vi "PicoScope3000aGetStreamingValues.vi"(9 "deviceIndex":u16, 11 "error in":errorcluster) -> (0 "Start Index":u32, 1 "Trigger":cluster{bool, "triggeredAt (Total samples)":u32}, 3 "error out":errorcluster, 4 "Number of Samples":i32, 5 "ready":i16, 6 "Auto Stopped":bool)   [LabVIEW 2010]
doc: "This VI is used in streaming mode to get the latest values from the driver. It should be called in a loop after the oscilloscope has been set up using PicoScope3000aSettings.vi and streaming has been started by calling PicoScope3000aStartStreaming.vi. The VI outputs the number of samples available and the start index of these samples in the array output by PicoScope3000aStartStreaming.vi."
uses:
  ps3000aWrap.dll
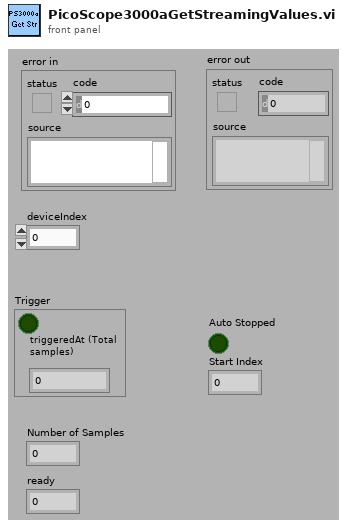
[diagram p1: front panel]
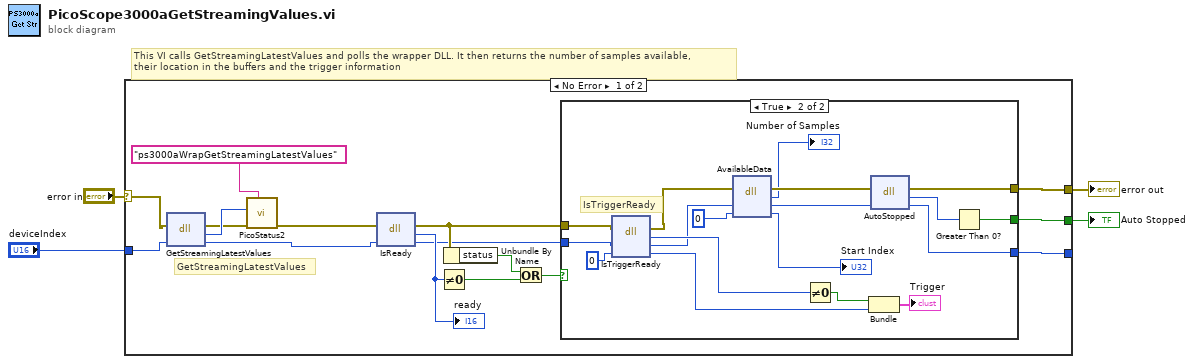
[diagram p0: block diagram]
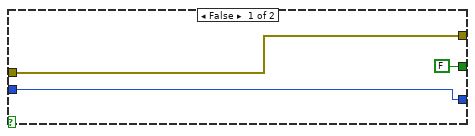
[diagram p2: hidden frame]
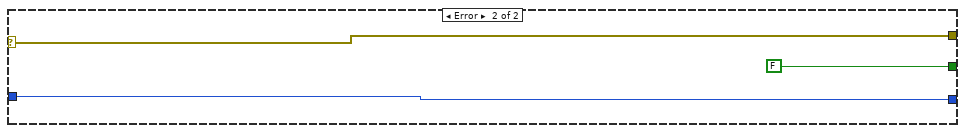
[diagram p3: hidden frame]
diagram:
  # "This VI calls GetStreamingLatestValues and polls the wrapper DLL. It then returns the number of samples available, \ntheir location in the buffers and the trigger information"
  n1 = case shown="No Error" "error in" {
    selector: "error in" -> [w14 w44]
    tunnel: [w20 w44] -> w3
    tunnel: [w19 w42] -> _
    tunnel: [w18 FALSE] -> w2
    tunnel: "deviceIndex" -> [w9 w42]
    frame No Error {
      # "GetStreamingLatestValues"
      n2 = dll-call lib="ps3000aWrap.dll" fn="GetStreamingLatestValues" ("PS5000.dll:_ps5000SetDataBuffer@16")(error in=w14, "deviceIndex"=w9) -> (error out=w7:errorcluster, "PICO_STATUS"=w8:u32, "deviceIndex"=w13:u16)  [unwired: 2 in, 1 out]
      n3 = call "PicoStatus2.vi"("PICO source"="ps3000aWrapGetStreamingLatestValues" ("source"), "Error in"=w7, "PICO STATUS"=w8) -> ("error out"=w5:errorcluster)  [unwired: 5 in, 1 out]
      n4 = dll-call lib="ps3000aWrap.dll" fn="IsReady" ("PS5000.dll:_ps5000SetDataBuffer@16")(error in=w5, "DeviceIndex"=w13) -> (error out=w12:errorcluster, "ready"=w11:i16, "DeviceIndex"=w10:u16)  [unwired: 2 in, 1 out]
      "ready" <- w11
      n5 = Not Equal To 0?(x=w11) -> (x != 0?=w16:bool)
      n6 = Unbundle By Name(w12) -> ("status"=w17:bool)
      n7 = Or(x=w17, y=w16) -> (x .or. y?=w15:bool)
      n8 = case shown="True" w15 {
        tunnel: [w23 w24] -> w20
        tunnel: w10 -> [w22 w37]
        tunnel: w12 -> [w23 w38]
        tunnel: [w22 w32] -> w19
        tunnel: [FALSE w39] -> w18
        frame False {
        }
        frame True {
          # "IsTriggerReady"
          n9 = dll-call lib="ps3000aWrap.dll" fn="IsTriggerReady" ("PS5000.dll:_ps5000SetDataBuffer@16")(error in=w38, "deviceIndex"=w37, "triggeredAt"=u32 0) -> (error out=w31:errorcluster, "triggered"=w34:i16, "deviceIndex"=w30:u16, "triggeredAt"=w35:u32)  [unwired: 2 in, 1 out]
          n10 = dll-call lib="ps3000aWrap.dll" fn="AvailableData" ("PS5000.dll:_ps5000Stop@4")(error in=w31, "deviceIndex"=w30, "startIndex"=u32 0) -> (error out=w28:errorcluster, "numSamples"=→"Number of Samples":i32, "deviceIndex"=w27:u16, "startIndex"=→"Start Index":u32)  [unwired: 2 in, 1 out]
          n11 = Not Equal To 0?(x=w34) -> (x != 0?=w41:bool)
          n12 = Bundle(w41, "triggeredAt"=w35) -> (→"Trigger":cluster{bool, "triggeredAt":u32})  [unwired: 1 in]
          n13 = dll-call lib="ps3000aWrap.dll" fn="AutoStopped"(error in=w28, "deviceIndex"=w27) -> (error out=w24:errorcluster, "AutoStopped"=w33:i16, "deviceIndex"=w32:u16)  [unwired: 2 in, 1 out]
          n14 = Greater Than 0?(x=w33) -> (x > 0?=w39:bool)
        }
      }
    }
    frame Error {
    }
  }
  "error out" <- w3
  "Auto Stopped" <- w2
